vi "Read Sweep Configuration File.vi"(8 "error in (no error)":errorcluster, 10 "Path":path, 11 "SweepControl in":refnum<class "SMO.SweepControl.lvclass">) -> (0 "error out":errorcluster, 2 "Data":variant, 3 "SweepControl out":refnum<class "SMO.SweepControl.lvclass">)   [LabVIEW 2019, in "SMO.SweepControl.lvclass"]
uses:
  SMO.SweepControl.lvclass
  Typedefs/Enum - Experiments.ctl
  Typedefs/Continuous B Sweep JSON--Cluster.ctl
  Typedefs/Enum - Priority.ctl
  Typedefs/Enum - Action.ctl
  Typedefs/Cluster - ScanControl.ctl
  Typedefs/ScanControl.ctl
  Typedefs/Cluster - ScanParamters.ctl
  Typedefs/ScanParamters.ctl
  Typedefs/Sweep Control JSON--Cluster.ctl
  <vilib>/addons/_JKI.lib/Serialization/JSON/JKI JSON Serialization.lvlib
  <userlib>/LevyLab/Krohn Hite 7008/typedefs/Input Configuration-Enum.ctl
  <userlib>/LevyLab/Krohn Hite 7008/Instrument.KH7008.lvclass
  <userlib>/LevyLab/Krohn Hite 7008/typedefs/Shunt-Enum.ctl
  <userlib>/LevyLab/Krohn Hite 7008/typedefs/Gain-Enum.ctl
  <userlib>/LevyLab/Krohn Hite 7008/typedefs/Channel-Enum.ctl
  Control Experiment/Typedefs/Wiring Description--v2--cluster.ctl
  Control Experiment/Control Experiment.lvclass
  Control Experiment/Typedefs/Experiment Description--cluster.ctl
  SMO.Transport/Typedefs/Lockin_Sweep JSON--Cluster.ctl
  SMO.Transport/SMO.Transport.lvclass
  <userlib>/LevyLab/Krohn Hite 7008/typedefs/Coupling-Enum.ctl
  <userlib>/LevyLab/Krohn Hite 7008/typedefs/Filter-Enum.ctl
  <userlib>/LevyLab/Krohn Hite 7008/typedefs/SetAll-Cluster.ctl
  <userlib>/LevyLab/Krohn Hite 7008/typedefs/SetAll-Array.ctl
  <userlib>/LevyLab/Lockin-Multichannel/Instrument.DAQ/Typedefs/REF.Channel--Cluster.ctl
  <userlib>/LevyLab/Lockin-Multichannel/Instrument.DAQ/Instrument.DAQ.lvclass
  <userlib>/LevyLab/Lockin-Multichannel/Instrument.DAQ/Typedefs/REF.Channel--Cluster--Array.ctl
  <userlib>/LevyLab/Lockin-Multichannel/Instrument.DAQ/Typedefs/AO.Channel.Function--Enum.ctl
  <userlib>/LevyLab/Lockin-Multichannel/Instrument.DAQ/Typedefs/AO.Channel--Cluster.ctl
  <userlib>/LevyLab/Lockin-Multichannel/Instrument.DAQ/Typedefs/AO.Channel--Cluster--Array.ctl
  Control Experiment/Typedefs/Instrument Types--combo.ctl
  Control Experiment/Typedefs/Instrument--enum.ctl
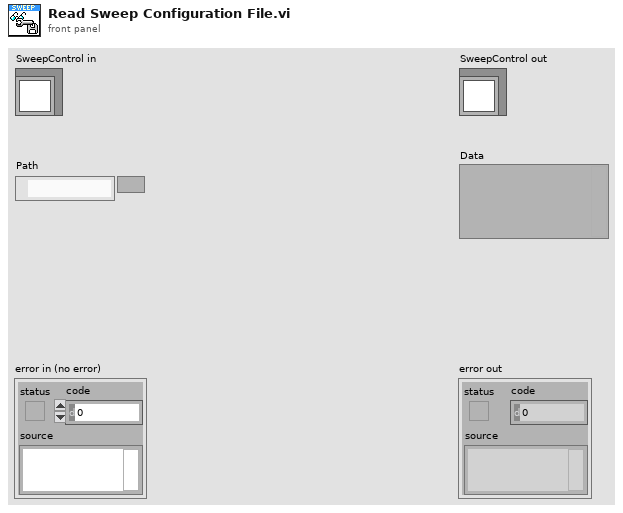
[diagram p1: front panel]
types:
  T1 = typedef "SMO.Transport.lvclass/Lockin_Sweep JSON--Cluster.ctl" = cluster{"Sweep Time (s)":dbl, "Sweep Start (V)":dbl, "Sweep End (V)":dbl, "Sweep Channel":i32}
  T2 = typedef "SMO.SweepControl.lvclass/Continuous B Sweep JSON--Cluster.ctl" = cluster{"Continuous B Sweep":cluster{"Experiment":T3, "B field values":dbl[]}, "Experiment Description":T4, "Wiring Configuration":T7, "Lockin":cluster{"Channels: AO":T8, "Channels: Lockin":T11}, "Krohn Hite":cluster{"Channel Setting":T13}}
  T3 = typedef "SMO.SweepControl.lvclass/Enum - Experiments.ctl" = enum16{"IV", "IV_Fast", "THz_DelayLine", "Lockin_Vsg", "Lockin_Sweep", "Lockin_Time", "AI WFM time", "Lockin (experimental)"}
  T4 = typedef "Control Experiment.lvclass/Experiment Description--cluster.ctl" = cluster{"User":string, "Device":string, "Device Path":path, "Device Description":string, "Experiment Path":path, "Experiment Description":string, "Instrument":T5, "Instruments":cluster{"class path":path, "Address":string, "Type":T6}[], "Sweep":cluster{"key":string, "value":variant}[]}
  T5 = typedef "Control Experiment.lvclass/Instrument--enum.ctl" = enum16{"----- AFM/EBL -----", "AGILENT", "CYPHER", "Gemini2", "JEOL", "MFP3D", "----- Cryostat -----", "CF900", "DR200", "MNK", "PPMS (simulated)", "PPMS 1", "PPMS 2", "PPMS 3", "----- Optics -----", "THz 1 (Element 2/Montana)", "THz 2 (Tsunami/Janis)"}
  T6 = typedef "Control Experiment.lvclass/Instrument Types--combo.ctl" = string
  T7 = typedef "Control Experiment.lvclass/Wiring Description--v2--cluster.ctl" = cluster{"AI":cluster{"Channel":u32, "Gain":dbl}, "Device":cluster{"Electrode":string, "Label":string, "Type":string}, "KH":cluster{"Channel":string, "Configuration":string, "Gain":u32, "Shunt Resistor":u32}, "AO":cluster{"Channel":u32, "Gain":dbl}}
  T8 = typedef "Instrument.DAQ.lvclass/AO.Channel--Cluster--Array.ctl" = T9[]
  T9 = typedef "Instrument.DAQ.lvclass/AO.Channel--Cluster.ctl" = cluster{"Enable?":bool, "Channel":i32, "Amplitude":dbl, "Offset":dbl, "Frequency":dbl, "Phase":dbl, "Function":T10, "Sweeping?":bool}
  T10 = typedef "Instrument.DAQ.lvclass/AO.Channel.Function--Enum.ctl" = enum16{"Sine", "Triangle", "Square"}
  T11 = typedef "Instrument.DAQ.lvclass/REF.Channel--Cluster--Array.ctl" = T12[]
  T12 = typedef "Instrument.DAQ.lvclass/REF.Channel--Cluster.ctl" = cluster{"Enable?":bool, "Channel":i32, "Frequency":dbl, "Phase":dbl, "TC":dbl, "Roll-Off":i32}
  T13 = typedef "Instrument.KH7008.lvclass/SetAll-Array.ctl" = T14[]
  T14 = typedef "Instrument.KH7008.lvclass/SetAll-Cluster.ctl" = cluster{"Channel":T15, "Gain":T16, "Bandwidth Filter":T17, "Shunt Resistor":T18, "Coupling":T19, "Input Config":T20}
  T15 = typedef "Instrument.KH7008.lvclass/Channel-Enum.ctl" = enum16{"Channel 1", "Channel 2", "Channel 3", "Channel 4", "Channel 5", "Channel 6", "Channel 7", "Channel 8"}
  T16 = typedef "Instrument.KH7008.lvclass/Gain-Enum.ctl" = enum16{"1x", "10x", "100x", "1000x"}
  T17 = typedef "Instrument.KH7008.lvclass/Filter-Enum.ctl" = enum16{"OFF", "ON"}
  T18 = typedef "Instrument.KH7008.lvclass/Shunt-Enum.ctl" = enum16{"Open", "50 Ohms", "500 Ohms", "5k Ohms", "50k Ohms", "10M Ohm"}
  T19 = typedef "Instrument.KH7008.lvclass/Coupling-Enum.ctl" = enum16{"AC", "DC"}
  T20 = typedef "Instrument.KH7008.lvclass/Input Configuration-Enum.ctl" = enum16{"Ground", "SE+ (-gnd)", "SE- (+gnd)", "Differential"}
  T21 = typedef "SMO.SweepControl.lvclass/Sweep Control JSON--Cluster.ctl" = cluster{"Experiment":T3, "Repeat Experiment":i32, "Scan control":T22, "Scan parameters":T26}
  T22 = typedef "SMO.SweepControl.lvclass/ScanControl.ctl" = T23[]
  T23 = typedef "SMO.SweepControl.lvclass/Cluster - ScanControl.ctl" = cluster{"Priority":T24, "Scan name":T25}
  T24 = typedef "SMO.SweepControl.lvclass/Enum - Priority.ctl" = enum16{"Priority 0", "Priority 1", "Priority 2", "Priority 3", "Priority 4", "Priority 5"}
  T25 = typedef "SMO.SweepControl.lvclass/Enum - Action.ctl" = enum16{"OFF", "time", "Lockin Amplitude", "Lockin Frequency", "Lockin Bias", "Delay", "Strain", "DAQ Bias", "Magnet Field", "Temperature", "MW f1", "MW f2", "MW Amplitude1", "MW Amplitude2"}
  T26 = typedef "SMO.SweepControl.lvclass/ScanParamters.ctl" = T27[]
  T27 = typedef "SMO.SweepControl.lvclass/Cluster - ScanParamters.ctl" = cluster{"Start":dbl, "End":dbl, "Step":dbl, "Rate":dbl, "Waveform type":enum16{"linear", "triangle", "power"}, "wait (ms or K)":dbl, "Address":string, "channel":i32}
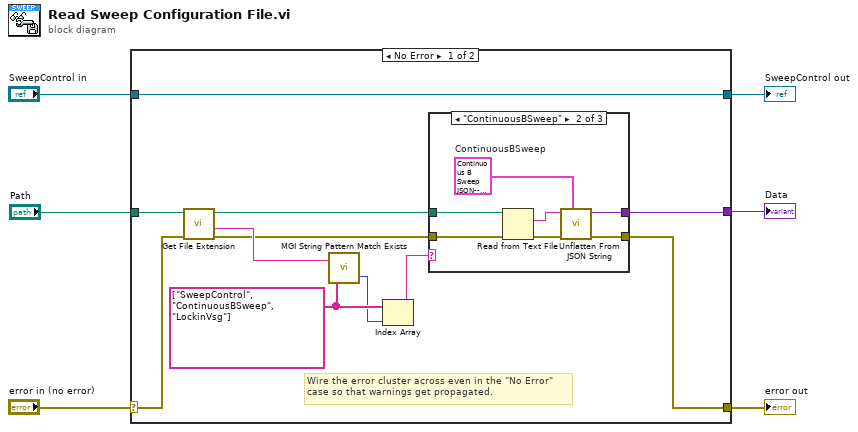
[diagram p0: block diagram]
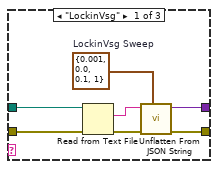
[diagram p2: hidden frame]
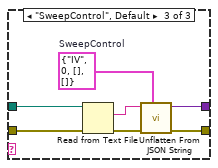
[diagram p3: hidden frame]
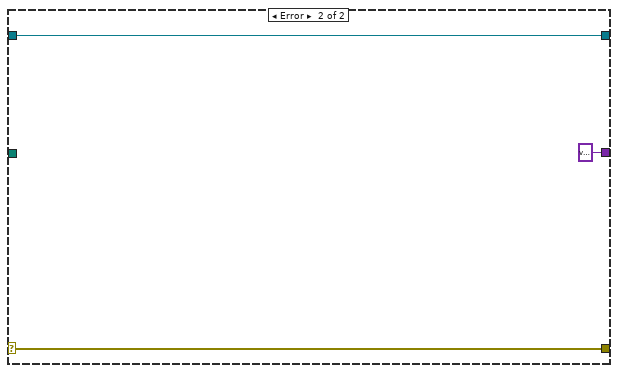
[diagram p4: hidden frame]
diagram:
  n1 = case shown="No Error" "error in (no error)" {
    selector: "error in (no error)" -> [w8 w41]
    tunnel: [w7 w41] -> w5
    tunnel: [w17 w40] -> w3
    tunnel: "SweepControl in" -> [w17 w40]
    tunnel: "Path" -> [w16 _]
    tunnel: [w9 variant ("Variant")] -> w1
    frame No Error {
      w14 = string[] ["SweepControl", "ContinuousBSweep", "LockinVsg"] ("Patterns to Try")
      # "Wire the error cluster across even in the \"No Error\"\ncase so that warnings get propagated."
      n2 = call <vilib>:"Get File Extension.vi"("error in (no error)"=w8, "file"=w16) -> ("error out"=w11:errorcluster, "filename without extension"=w13:string, "dup file"=w10:path)  [unwired: 5 in, 2 out]
      n3 = call <userlib>:"MGI String Pattern Match Exists.vi"("Patterns to Try"=w14, "String"=w13) -> ("Index of First Pattern Matched"=w12:i32)  [unwired: 1 out]
      n4 = Index Array(array=w14, index=w12) -> (element=w15:string)
      n5 = case shown="\"ContinuousBSweep\"" w15 {
        tunnel: w11 -> [w22 w29 w36]
        tunnel: w10 -> [w21 w28 w35]
        tunnel: [w19 w27 w34] -> w9
        tunnel: [w18 w26 w33] -> w7
        frame "LockinVsg" {
          w20 = T1 {"Sweep Time (s)"=0.001, "Sweep Start (V)"=0.0, "Sweep End (V)"=0.1, "Sweep Channel"=1}  # LockinVsg Sweep
          n6 = Read from Text File(file (use dialog)=w21, error in=w22) -> (text=w23:string, error out=w24:errorcluster)  [unwired: 2 in, 2 out]
          n7 = call <vilib>:"Unflatten From JSON String.vi"("Type and Defaults"=w20, "error in (no error)"=w24, "JSON String"=w23) -> ("error out"=w18:errorcluster, "Variant"=w19:variant)  [unwired: 7 in]
        }
        frame "ContinuousBSweep" {
          w25 = T2 {"Continuous B Sweep"={"Experiment"=enum."IV", "B field values"=[]}, "Experiment Description"={"User"="", "Device"="", "Device Path"=path "", "Device Description"="", "Experiment Path"=path "", "Experiment Description"="", "Instrument"=enum."PPMS 1", "Instruments"=[], "Sweep"=[]}, "Wiring Configuration"={"AI"={"Channel"=0, "Gain"=0.0}, "Device"={"Electrode"="", "Label"="", "Type"=""}, "KH"={"Channel"="", "Configuration"="", "Gain"=0, "Shunt Resistor"=0}, "AO"={"Channel"=0, "Gain"=0.0}}, "Lockin"={"Channels: AO"=[], "Channels: Lockin"=[]}, "Krohn Hite"={"Channel Setting"=[]}}  # ContinuousBSweep
          n8 = Read from Text File(file (use dialog)=w28, error in=w29) -> (text=w30:string, error out=w31:errorcluster)  [unwired: 2 in, 2 out]
          n9 = call <vilib>:"Unflatten From JSON String.vi"("Type and Defaults"=w25, "error in (no error)"=w31, "JSON String"=w30) -> ("error out"=w26:errorcluster, "Variant"=w27:variant)  [unwired: 7 in]
        }
        frame "SweepControl", Default {
          w32 = T21 {"Experiment"=enum."IV", "Repeat Experiment"=0, "Scan control"=[], "Scan parameters"=[]}  # SweepControl
          n10 = Read from Text File(file (use dialog)=w35, error in=w36) -> (text=w37:string, error out=w38:errorcluster)  [unwired: 2 in, 2 out]
          n11 = call <vilib>:"Unflatten From JSON String.vi"("Type and Defaults"=w32, "error in (no error)"=w38, "JSON String"=w37) -> ("error out"=w33:errorcluster, "Variant"=w34:variant)  [unwired: 7 in]
        }
      }
    }
    frame Error {
    }
  }
  "error out" <- w5
  "SweepControl out" <- w3
  "Data" <- w1
